vi "ReadGlobalStop.vi"() -> (0 "Global DataPacker Stop":bool)   [LabVIEW 2018, in "feGEM DataPacker.lvlib"]
uses:
  feGEM DataPacker.lvlib
  DataPacker_Global_Stop_Enum.ctl
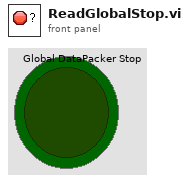
[diagram p1: front panel]
types:
  T1 = typedef "feGEM DataPacker.lvlib/DataPacker_Global_Stop_Enum.ctl" = enum16{"Reset", "Set Soft Stop", "Get Soft Stop", "Set Hard Stop", "Get Hard Stop", "Get Any Stop"}
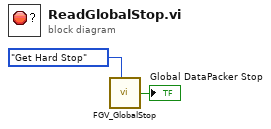
[diagram p0: block diagram]
diagram:
  n1 = call "FGV_GlobalStop.vi"("Enum"=DataPacker_Global_Stop_Enum."Get Hard Stop") -> ("Stop"=→"Global DataPacker Stop":bool)  [unwired: 4 in]
